vi "Setup Statically-Linked subWorkers.vi"(8 "error in":errorcluster, 11 "First Level Worker in":refnum<class "First Level Worker.lvclass">) -> (0 "error out":errorcluster, 3 "First Level Worker out":refnum<class "First Level Worker.lvclass">)   [LabVIEW 2017, in "Method 2.lvlib" / "First Level Worker.lvclass"]
doc: "This VI performs a setup of all the statically-linked subWorkers that belong to the Worker that owns this VI. This VI must be called <b>before</b> any statically-linked subWorkers are called."
uses:
  First Level Worker.lvclass
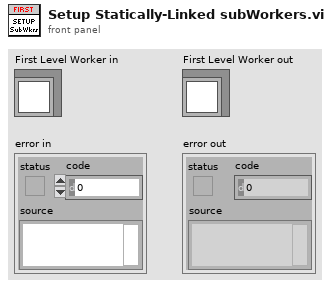
[diagram p1: front panel]
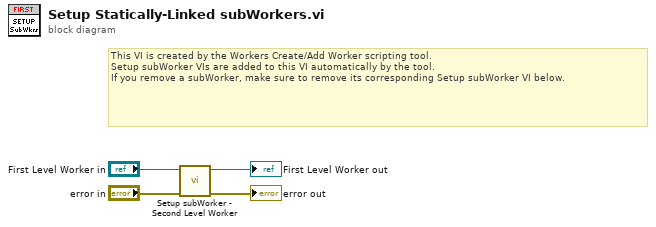
[diagram p0: block diagram]
diagram:
  # "This VI is created by the Workers Create/Add Worker scripting tool.\nSetup subWorker VIs are added to this VI automatically by the tool.\nIf you remove a subWorker, make sure to remove its corresponding Setup subWorker VI below."
  n1 = call "Setup subWorker - Second Level Worker.vi"("error in"="error in", "First Level Worker in"="First Level Worker in") -> ("error out"=→"error out":errorcluster, "First Level Worker out"=→"First Level Worker out":refnum<class "First Level Worker.lvclass">)  [unwired: 8 in]
